vi "Read TDMS Comments.vi"(8 "error in (no error)":errorcluster, 11 "path":path) -> (0 "error out":errorcluster, 2 "Notes":string)   [LabVIEW 2016, in "Data.TDMS.lvclass"]
uses:
  Data.TDMS.lvclass
panel:
  out "file path out":path
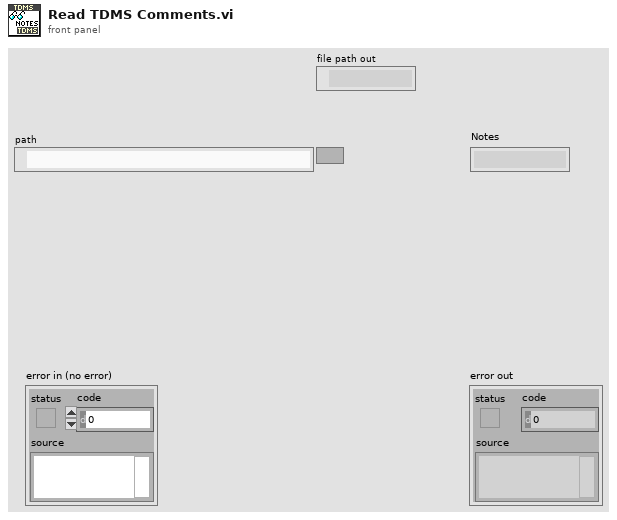
[diagram p1: front panel]
types:
  T1 = enum16{"open", "open or create", "create or replace", "create", "open (read-only)"}
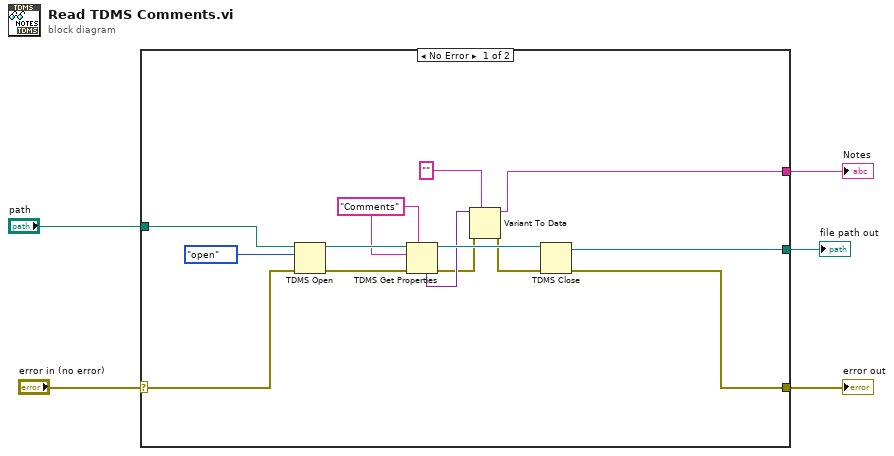
[diagram p0: block diagram]
diagram:
  n1 = case shown="No Error" "error in (no error)" {
    selector: "error in (no error)" -> [w13 w20]
    tunnel: [w16 w20] -> w4
    tunnel: "path" -> [w15 _]
    tunnel: [w7 _] -> w2
    tunnel: [w6 _] -> w1
    frame No Error {
      w12 = "Comments" ("group name")
      n2 = TDMS Open(8:w13, 10:T1."open" ("operation (0:open)"), 11:w15) -> (0:w17:errorcluster, 3:w18:refnum<k34>)  [unwired: 4 in]
      n3 = TDMS Get Properties(7:w12, 8:w17, 10:w12, 11:w18) -> (0:w9:errorcluster, 3:w14:refnum<k34>, 4:w11:variant)  [unwired: 2 in, 3 out]
      n4 = Variant To Data(error in=w9, type="" ("group name"), Variant=w11) -> (data=w7:string, error out=w8:errorcluster)
      n5 = TDMS Close(8:w8, 11:w14) -> (0:w16:errorcluster, 3:w6:path)
    }
    frame Error {
    }
  }
  "error out" <- w4
  "Notes" <- w2
  "file path out" <- w1
